vi "IFNoise-Plot.vi"(0 "Runtime":T1, 7 "Mic signal":dbl[](array[numeric]), 11 "error in (no error)":errorcluster, 12 "Acquired":i32) -> (4 "Mags":cluster{"Frequency (Hz)":dbl[], "dB":dbl[]}[](array[cluster]), 8 "Time":cluster{i32, "dx":dbl, "Array":dbl[]}, 14 "dB SPL":dbl, 15 "error out":errorcluster)   [LabVIEW 2015]
uses:
  Type Defs/IFNoise-Runtime.ctl
  Utility VIs/Math VIs/Linear to dB (scalar).vi
  Utility VIs/Conversion VIs/Create Waveform Cluster (1D).vi
  Utility VIs/Math VIs/Linear to dB (array).vi
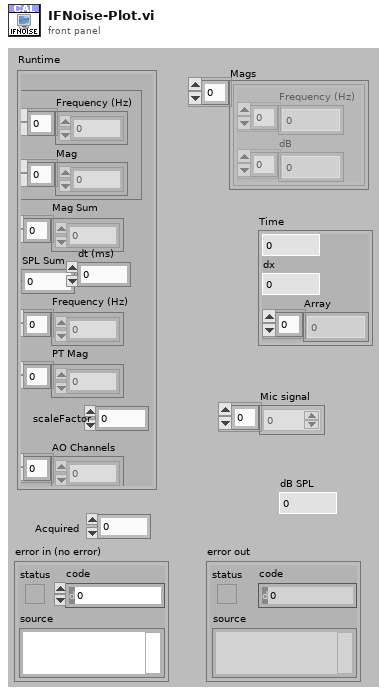
[diagram p1: front panel]
types:
  T1 = typedef "IFNoise-Runtime.ctl" = cluster{"Calibration":cluster{"Frequency (Hz)":dbl[], "Mag":dbl[]}, "Mag Sum":dbl[], "SPL Sum":dbl, "Frequency (Hz)":dbl[], "PT Mag":dbl[], "dt (ms)":dbl, "AO Channels":i32[], "scaleFactor":dbl}
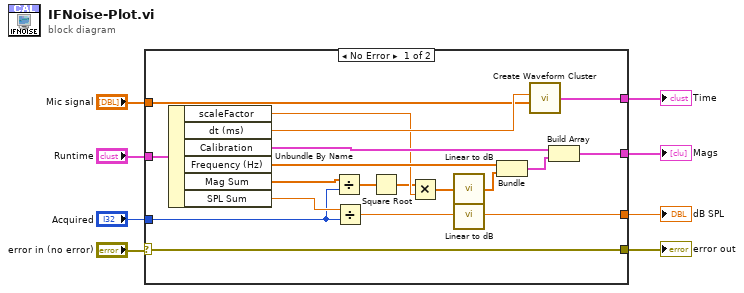
[diagram p0: block diagram]
diagram:
  n1 = case shown="No Error" "error in (no error)" {
    selector: "error in (no error)" -> [w27 w28]
    tunnel: [w27 w28] -> w7
    tunnel: "Runtime" -> [w26 _]
    tunnel: "Acquired" -> [w16 _]
    tunnel: [w21 _] -> w4
    tunnel: "Mic signal" -> [w19 _]
    tunnel: [w18 _] -> w2
    tunnel: [w14 _] -> w1
    frame No Error {
      n2 = Unbundle By Name(w26) -> ("scaleFactor"=w12:dbl, "dt (ms)"=w20:dbl, "Calibration"=w23:cluster{"Frequency (Hz)":dbl[], "Mag":dbl[]}, "Frequency (Hz)"=w25:dbl[], "Mag Sum"=w11:dbl[], "SPL Sum"=w17:dbl)
      n3 = Divide(x=w11, y=w16) -> (x/y=w10:dbl[])
      n4 = Divide(x=w17, y=w16) -> (x/y=w15:dbl)
      n5 = Square Root(x=w10) -> (sqrt(x)=w9:dbl[])
      n6 = Multiply(x=w9, y=w12) -> (x*y=w13:dbl[])
      n7 = call-poly "Linear to dB.vi"("linear"=w13) -> ("dB"=w24:dbl[])
      n8 = call-poly "Linear to dB.vi"("Linear"=w15) -> ("dB"=w14:dbl)
      n9 = Bundle("Frequency (Hz)"=w25, "dB"=w24) -> (w22:cluster{"Frequency (Hz)":dbl[], "dB":dbl[]})  [unwired: 1 in]
      n10 = call-poly "Create Waveform Cluster.vi"("Array"=w19, "dx"=w20) -> ("waveform cluster"=w18:cluster{i32, "dx":dbl, "Array":dbl[]})  [unwired: 2 in]
      n11 = Build Array(w23, w22) -> (w21:cluster{"Frequency (Hz)":dbl[], "dB":dbl[]}[])
    }
    frame Error {
    }
  }
  "error out" <- w7
  "Mags" <- w4
  "Time" <- w2
  "dB SPL" <- w1
